vi "Get Dev Screen Size.vi"(11 "screen size":T1(ring)) -> (2 "Max Row number":u8, 3 "Max Column number":u8)   [LabVIEW 2017, in "HD44780.lvclass"]
uses:
  HD44780.lvclass
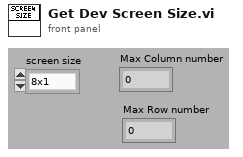
[diagram p1: front panel]
types:
  T1 = enum8{"8x1", "8x2", "12x4", "16x1", "16x2", "16x4", "20x1", "20x2", "20x4", "24x1", "24x2", "40x2", "40x4"}
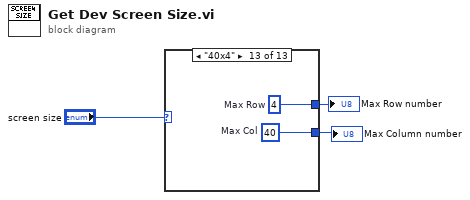
[diagram p0: block diagram]
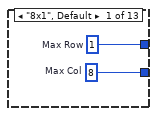
[diagram p2: hidden frame]
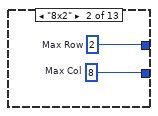
[diagram p3: hidden frame]
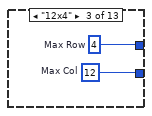
[diagram p4: hidden frame]
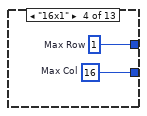
[diagram p5: hidden frame]
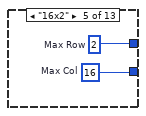
[diagram p6: hidden frame]
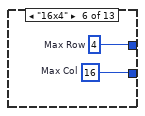
[diagram p7: hidden frame]
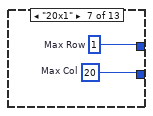
[diagram p8: hidden frame]
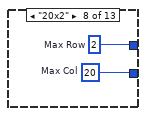
[diagram p9: hidden frame]
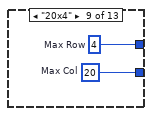
[diagram p10: hidden frame]
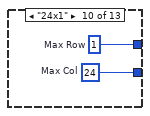
[diagram p11: hidden frame]
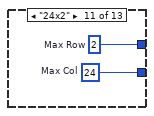
[diagram p12: hidden frame]
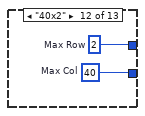
[diagram p13: hidden frame]
diagram:
  n1 = case shown="\"40x4\"" "screen size" {
    tunnel: [w5 w7 w9 w11 w13 w15 w17 w19 w21 w23 w25 w27 w29] -> w2
    tunnel: [w4 w6 w8 w10 w12 w14 w16 w18 w20 w22 w24 w26 w28] -> w3
    frame "8x1", Default {
      w4 = u8 8  # Max Col
      w5 = u8 1  # Max Row
    }
    frame "8x2" {
      w6 = u8 8  # Max Col
      w7 = u8 2  # Max Row
    }
    frame "12x4" {
      w8 = u8 12  # Max Col
      w9 = u8 4  # Max Row
    }
    frame "16x1" {
      w10 = u8 16  # Max Col
      w11 = u8 1  # Max Row
    }
    frame "16x2" {
      w12 = u8 16  # Max Col
      w13 = u8 2  # Max Row
    }
    frame "16x4" {
      w14 = u8 16  # Max Col
      w15 = u8 4  # Max Row
    }
    frame "20x1" {
      w16 = u8 20  # Max Col
      w17 = u8 1  # Max Row
    }
    frame "20x2" {
      w18 = u8 20  # Max Col
      w19 = u8 2  # Max Row
    }
    frame "20x4" {
      w20 = u8 20  # Max Col
      w21 = u8 4  # Max Row
    }
    frame "24x1" {
      w22 = u8 24  # Max Col
      w23 = u8 1  # Max Row
    }
    frame "24x2" {
      w24 = u8 24  # Max Col
      w25 = u8 2  # Max Row
    }
    frame "40x2" {
      w26 = u8 40  # Max Col
      w27 = u8 2  # Max Row
    }
    frame "40x4" {
      w28 = u8 40  # Max Col
      w29 = u8 4  # Max Row
    }
  }
  "Max Row number" <- w2
  "Max Column number" <- w3
